vi "particle_analysis.vi"() -> ()   [LabVIEW 2011]
panel:
  in  "Reset":bool
  in  "Enable":bool=TRUE
  out "Filename Out":path
  out "Saving Data":bool
  in  "stop":bool
  in  "Range (Threshold 1)":cluster{"Lower value":sgl, "Upper value":sgl}={"Lower value"=0.0, "Upper value"=109.0}
  out "error out":errorcluster
  in  "delay":dbl
  in  "error in":errorcluster
  out "Image Out":T1(plugin-control)
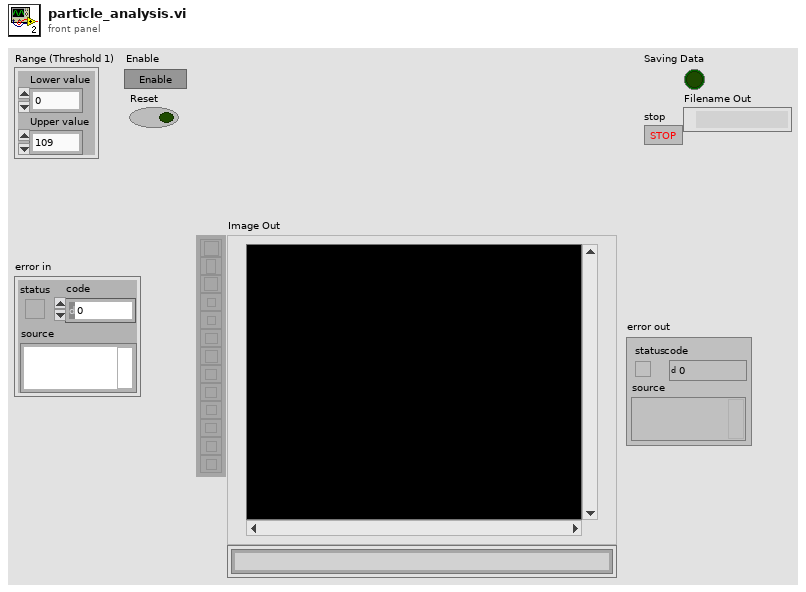
[diagram p1: front panel]
types:
  T1 = typedef "IMAQ Image.ctl" = refnum<image>
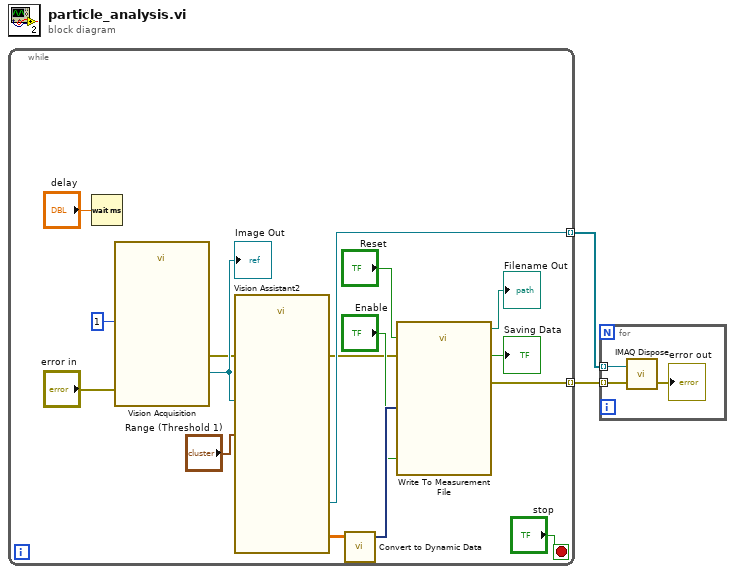
[diagram p0: block diagram]
diagram:
  n1 = while {
    tunnel: [w14] -> w2 mode=indexing
    tunnel: [w3] -> w1 mode=indexing
    stop <- "stop" stop-if-true
    n2 = Wait (ms)(milliseconds to wait="delay") -> ()  [unwired: 1 out]
    n3 = call "Vision Acquisition"("Number of Images"=1, "error in"="error in") -> ("Image Out"=w18:T1, "error out"=w17:errorcluster)  [unwired: 23 in, 1 out]
    "Image Out" <- w18
    n4 = call "Vision Assistant2"("Image In"=w18, "Range (Threshold 1)"="Range (Threshold 1)", "error in"=w17) -> ("Image Out"=w14:T1, "Particle Measurements (Pixels) (Particle Analysis 1)"=w10:dbl[][], "error out"=w4:errorcluster)  [unwired: 21 in, 1 out]
    n5 = call "Convert to Dynamic Data"("2D Array"=w10) -> ("Dynamic Data Type"=w9:dynamicdata)  [unwired: 3 in]
    n6 = call "Write To Measurement File"("Signals"=w9, "Reset"="Reset", "Enable"="Enable", "error in (no error)"=w4) -> ("Filename Out"=→"Filename Out":path, "Saving Data"=→"Saving Data":bool, "error out"=w3:errorcluster)  [unwired: 13 in]
  }
  n7 = for {
    tunnel: w2 -> [w21] mode=indexing
    tunnel: w1 -> [w20] mode=indexing
    n8 = call "IMAQ Dispose"("Image"=w21, "error in (no error)"=w20) -> ("error out"=→"error out":errorcluster)  [unwired: 4 in]
  }
